vi "Generic command handler.vi"(8 "error in (no error)":errorcluster, 10 "Message in":refnum<class "GenericMessage.lvclass">, 11 "AOTF in":refnum<class "Invivo_AOTF.lvclass">) -> (0 "error out":errorcluster, 2 "command":string, 3 "AOTF out":refnum<class "Invivo_AOTF.lvclass">)   [LabVIEW 2012, in "Invivo_AOTF.lvclass"]
doc: "The generic_command_handler processes the command 'generic'. Commands which are not part of the predefined list of commands fall under the 'generic' command for special activity."
uses:
  Invivo_AOTF.lvclass
  <vilib>/Distrio/Murmex/GenericMessage/GenericMessage.lvclass
  <vilib>/Distrio/Murmex/Murmex/Murmex.lvclass
panel:
  # "This method is called when the GENERIC\ntrigger is sent. \n\nOverride this method when your component needs to\nrespond to this trigger. \n\nCall parent for proper implementation"
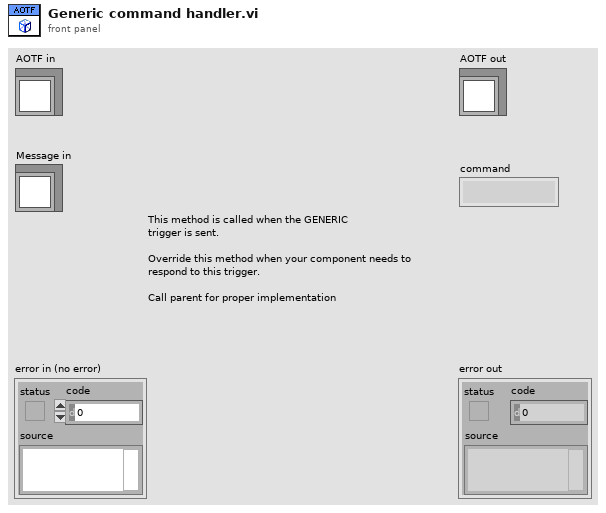
[diagram p1: front panel]
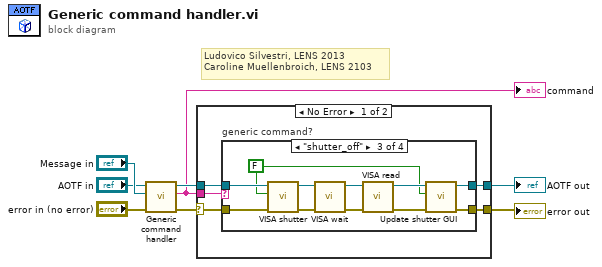
[diagram p0: block diagram]
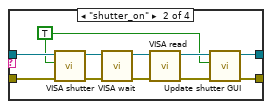
[diagram p3: hidden frame]
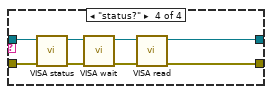
[diagram p4: hidden frame]
diagram:
  # "Ludovico Silvestri, LENS 2013\nCaroline Muellenbroich, LENS 2103"
  n1 = call-parent "Generic command handler.vi"("error in (no error)"="error in (no error)", "Message in"="Message in", "Murmex in"="AOTF in") -> ("error out"=w5:errorcluster, "value"=w1:string, "Murmex out"=w3:refnum<class "Invivo_AOTF.lvclass">)  [unwired: 6 in]
  "command" <- w1
  n2 = case shown="No Error" w5 {
    selector: w5 -> [w12 w46]
    tunnel: [w13 w46] -> w4
    tunnel: w3 -> [w11 w47]
    tunnel: [w10 w47] -> w2
    tunnel: w1 -> [w9 _]
    frame No Error {
      n3 = case "generic command?" shown="\"shutter_off\"" w9 {
        tunnel: [w14 w19 w30 w39] -> w13
        tunnel: w12 -> [w14 w26 w37 w44]
        tunnel: w11 -> [w15 w25 w36 w45]
        tunnel: [w15 w18 w31 w40] -> w10
        frame Default {
        }
        frame "shutter_on" {
          w16 = TRUE ("button::shutter")
          n4 = call-dynamic "VISA shutter.vi"("error in (no error)"=w26, "button::shutter"=w16, "AOTF in"=w25) -> ("error out"=w21:errorcluster, "AOTF out"=w24:refnum<class "Invivo_AOTF.lvclass">)  [unwired: 7 in]
          n5 = call-dynamic "VISA wait.vi"("error in (no error)"=w21, "AOTF in"=w24) -> ("error out"=w22:errorcluster, "AOTF out"=w23:refnum<class "Invivo_AOTF.lvclass">)  [unwired: 8 in]
          n6 = call-dynamic "VISA read.vi"("error in (no error)"=w22, "AOTF in"=w23) -> ("error out"=w20:errorcluster, "AOTF out"=w17:refnum<class "Invivo_AOTF.lvclass">)  [unwired: 7 in, 1 out]
          n7 = call-dynamic "Update shutter GUI.vi"("error in (no error)"=w20, "shutter on/off"=w16, "AOTF in"=w17) -> ("error out"=w19:errorcluster, "AOTF out"=w18:refnum<class "Invivo_AOTF.lvclass">)  [unwired: 7 in]
        }
        frame "shutter_off" {
          w27 = FALSE ("button::shutter")
          n8 = call-dynamic "VISA shutter.vi"("error in (no error)"=w37, "button::shutter"=w27, "AOTF in"=w36) -> ("error out"=w32:errorcluster, "AOTF out"=w35:refnum<class "Invivo_AOTF.lvclass">)  [unwired: 7 in]
          n9 = call-dynamic "VISA wait.vi"("error in (no error)"=w32, "AOTF in"=w35) -> ("error out"=w33:errorcluster, "AOTF out"=w34:refnum<class "Invivo_AOTF.lvclass">)  [unwired: 8 in]
          n10 = call-dynamic "VISA read.vi"("error in (no error)"=w33, "AOTF in"=w34) -> ("error out"=w29:errorcluster, "AOTF out"=w28:refnum<class "Invivo_AOTF.lvclass">)  [unwired: 7 in, 1 out]
          n11 = call-dynamic "Update shutter GUI.vi"("error in (no error)"=w29, "shutter on/off"=w27, "AOTF in"=w28) -> ("error out"=w30:errorcluster, "AOTF out"=w31:refnum<class "Invivo_AOTF.lvclass">)  [unwired: 7 in]
        }
        frame "status?" {
          n12 = call-dynamic "VISA status.vi"("error in (no error)"=w44, "AOTF in"=w45) -> ("error out"=w42:errorcluster, "AOTF out"=w43:refnum<class "Invivo_AOTF.lvclass">)  [unwired: 8 in]
          n13 = call-dynamic "VISA wait.vi"("error in (no error)"=w42, "AOTF in"=w43) -> ("error out"=w38:errorcluster, "AOTF out"=w41:refnum<class "Invivo_AOTF.lvclass">)  [unwired: 8 in]
          n14 = call-dynamic "VISA read.vi"("error in (no error)"=w38, "AOTF in"=w41) -> ("error out"=w39:errorcluster, "AOTF out"=w40:refnum<class "Invivo_AOTF.lvclass">)  [unwired: 7 in, 1 out]
        }
      }
    }
    frame Error {
    }
  }
  "error out" <- w4
  "AOTF out" <- w2
